vi "iPSread.vi"(8 "error in (no error)":errorcluster, 10 "iPSreadCtrl":T1=enum."Switch Heater Temp", 11 "VISA resource name":refnum<visa-resource-name>) -> (0 "error out":errorcluster, 1 "read buffer":string, 2 "number":dbl, 3 "VISA resource name out":refnum<visa-resource-name>)   [LabVIEW 2017]
uses:
  controls/iPSreadCtrl.ctl
  <vilib>/regexp/Match Regular Expression.xnode
panel:
  out "after match":string
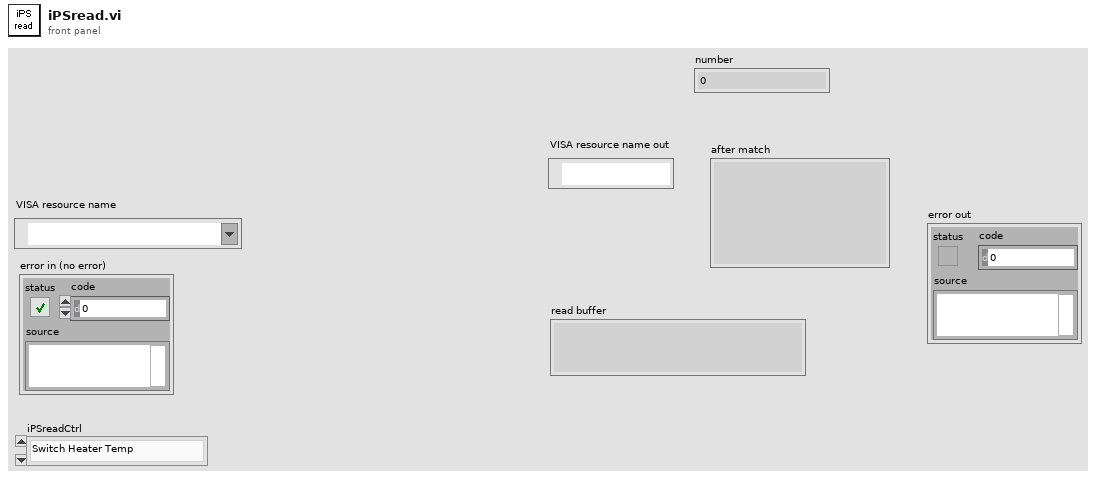
[diagram p1: front panel]
types:
  T1 = typedef "iPSreadCtrl.ctl" = enum16{"OutputField", "MagnetField", "Switch Heater Temp", "Field Rate", "Magnet Temp", "OutputVoltage"}
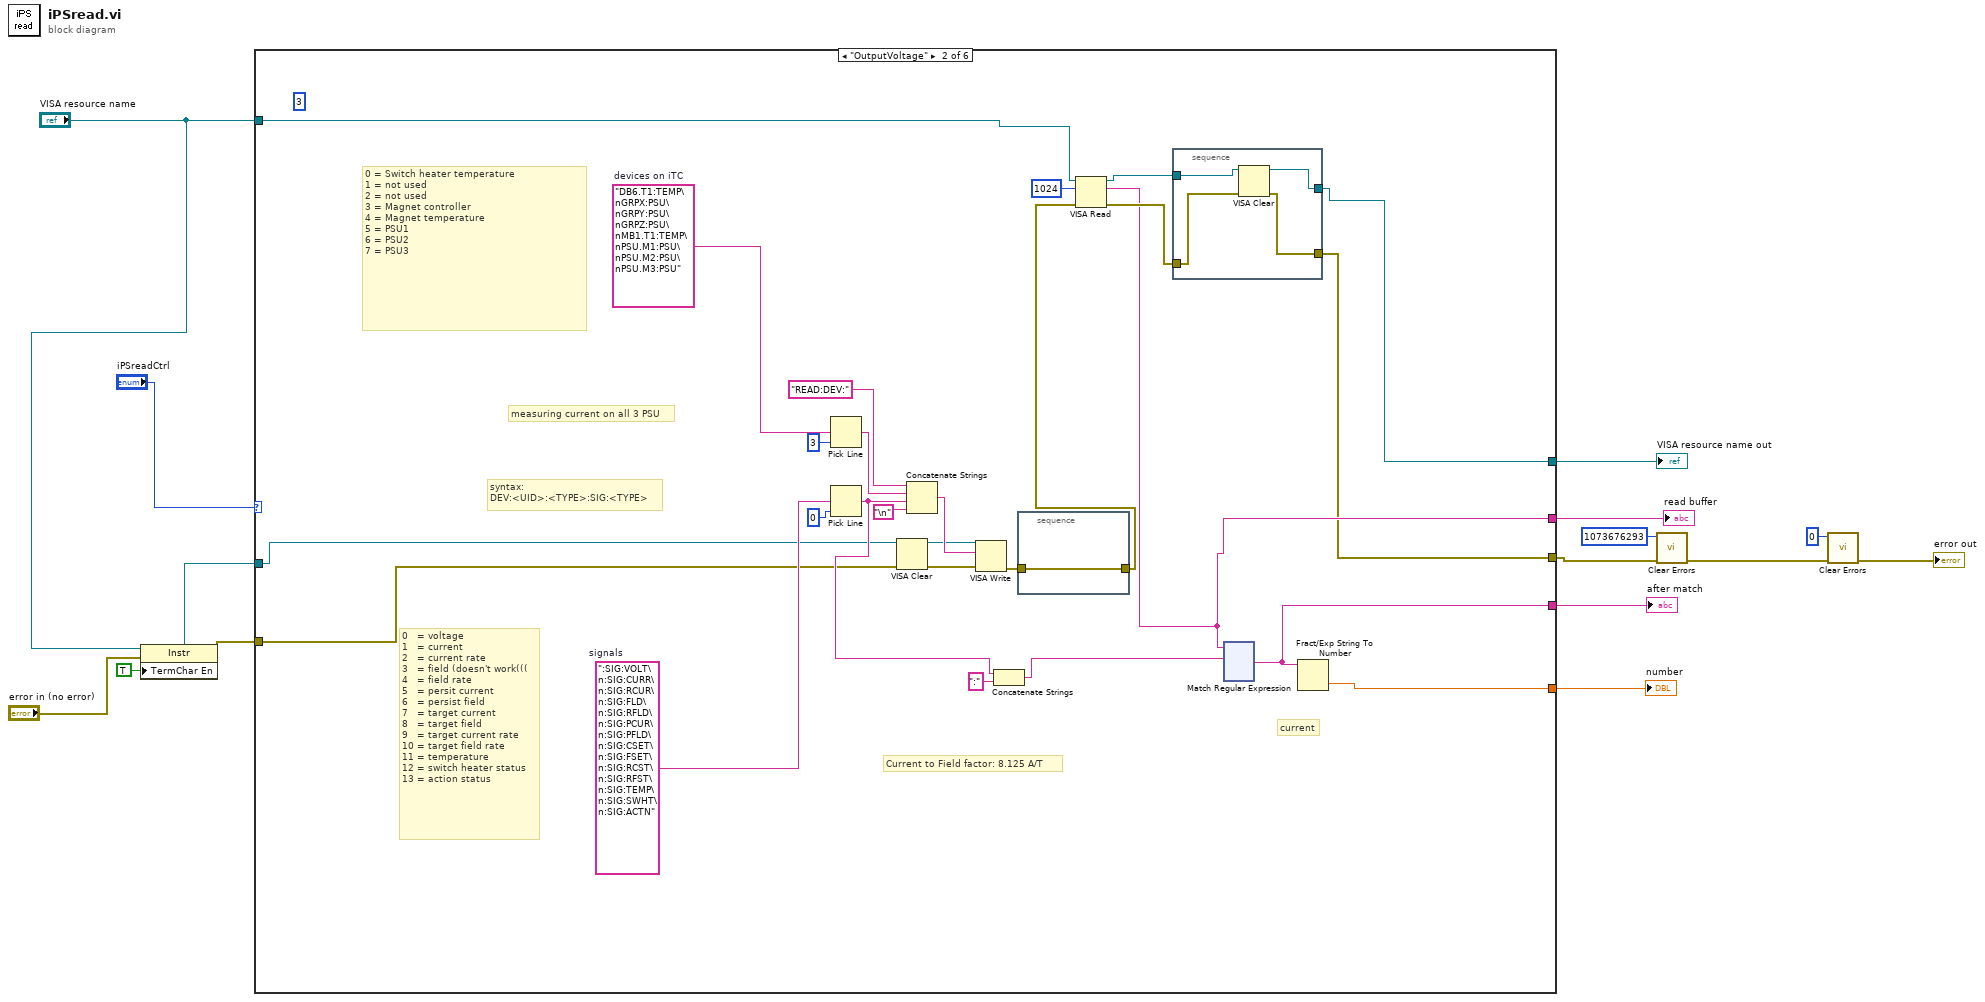
[diagram p0: block diagram]
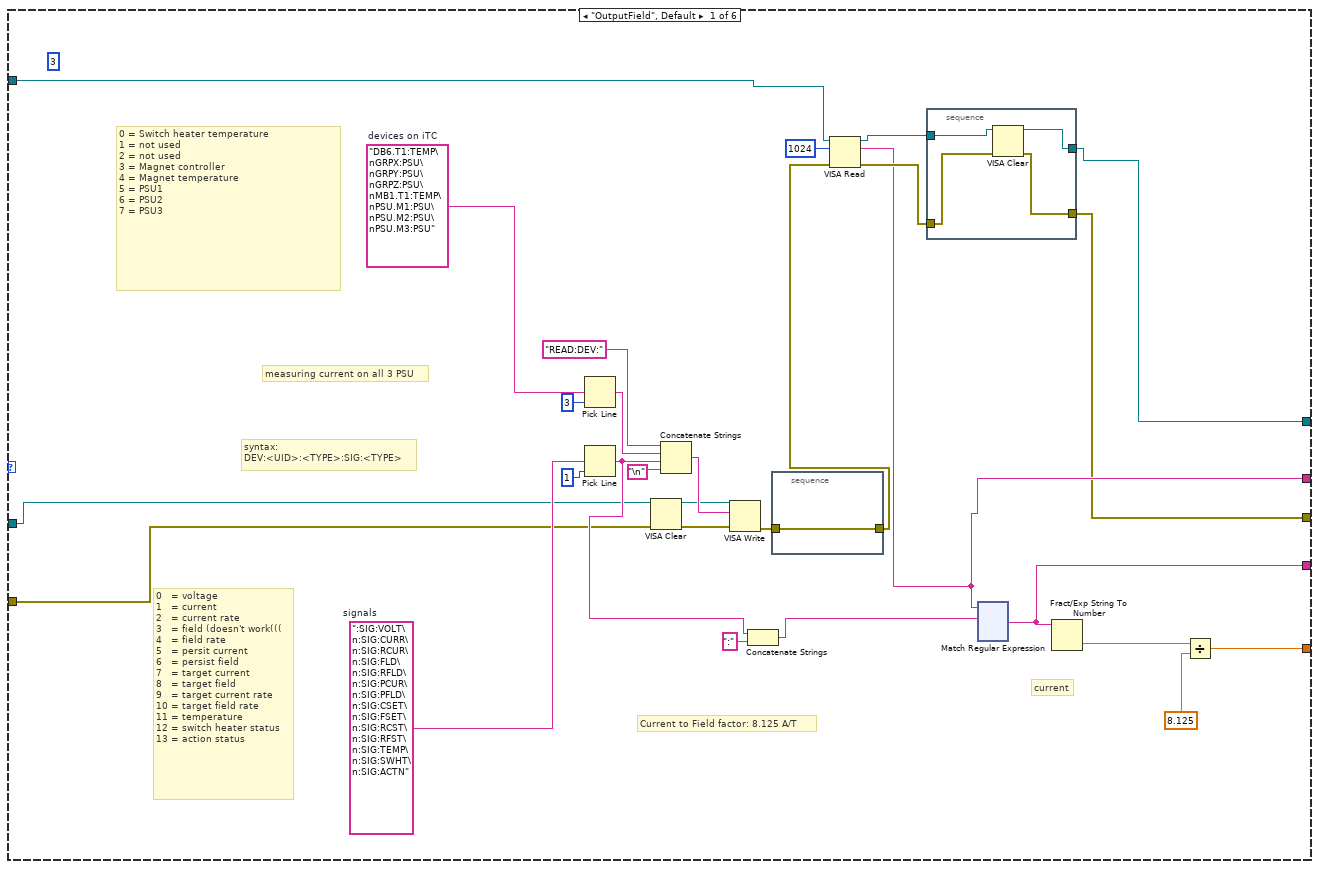
[diagram p2: hidden frame]
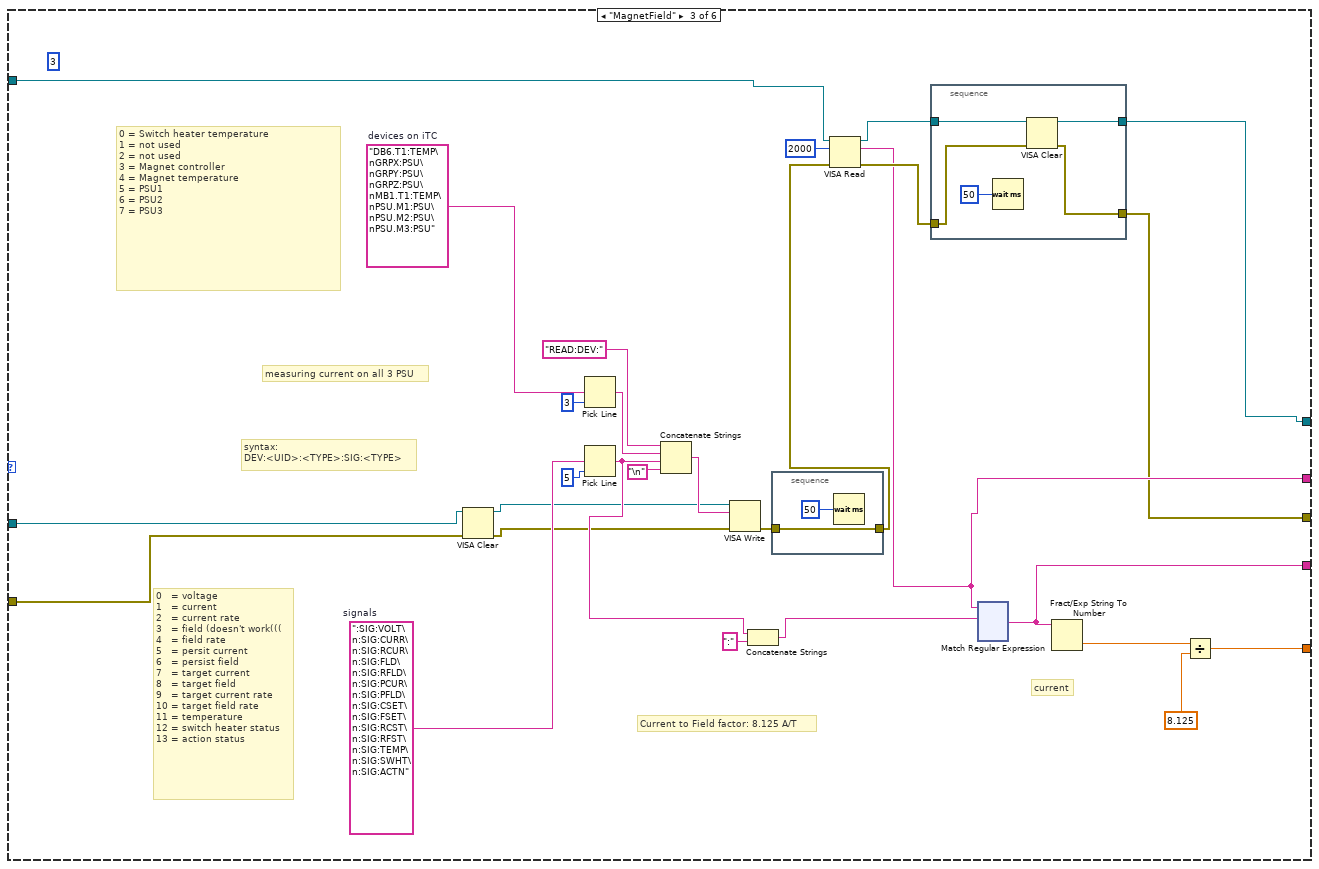
[diagram p3: hidden frame]
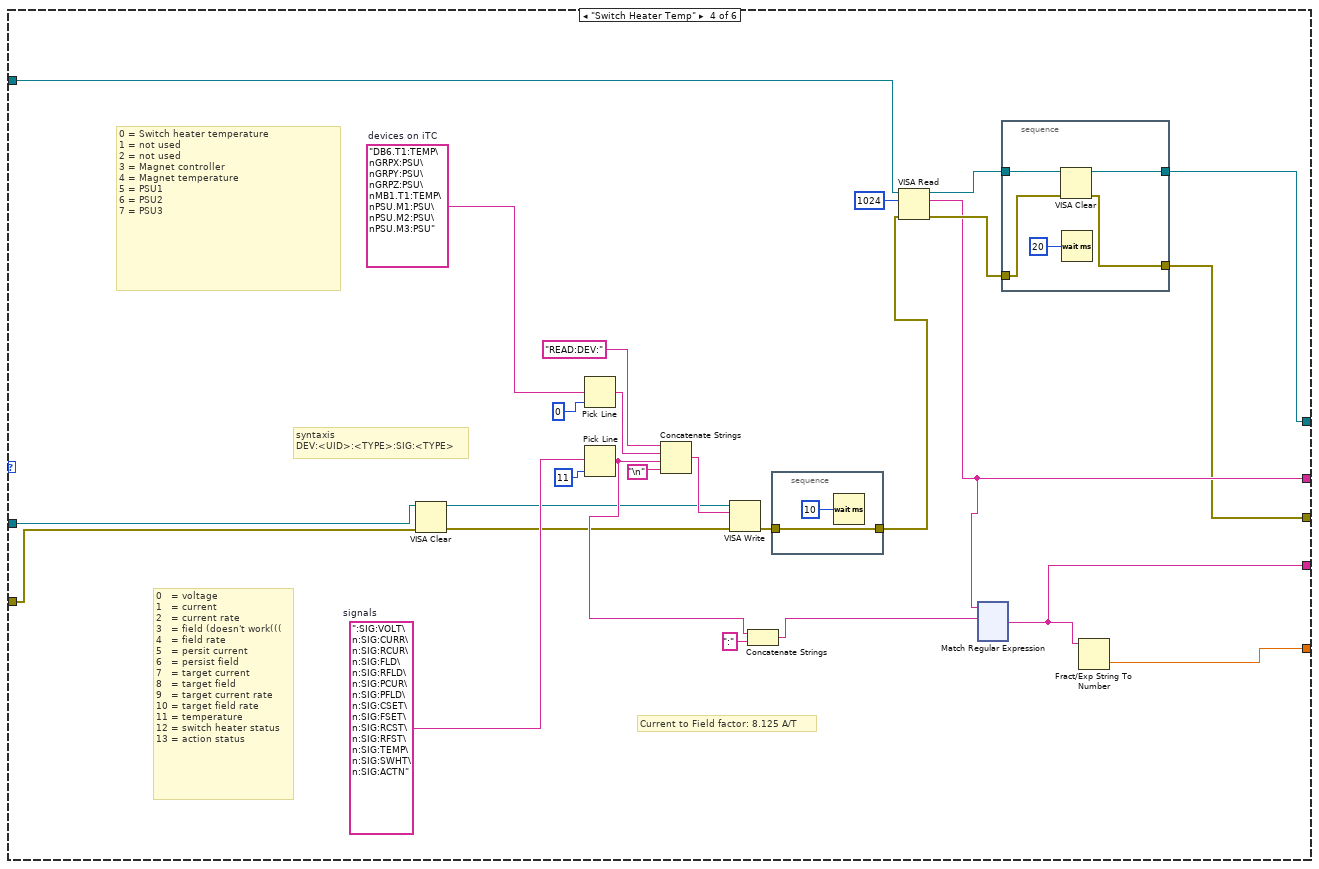
[diagram p4: hidden frame]
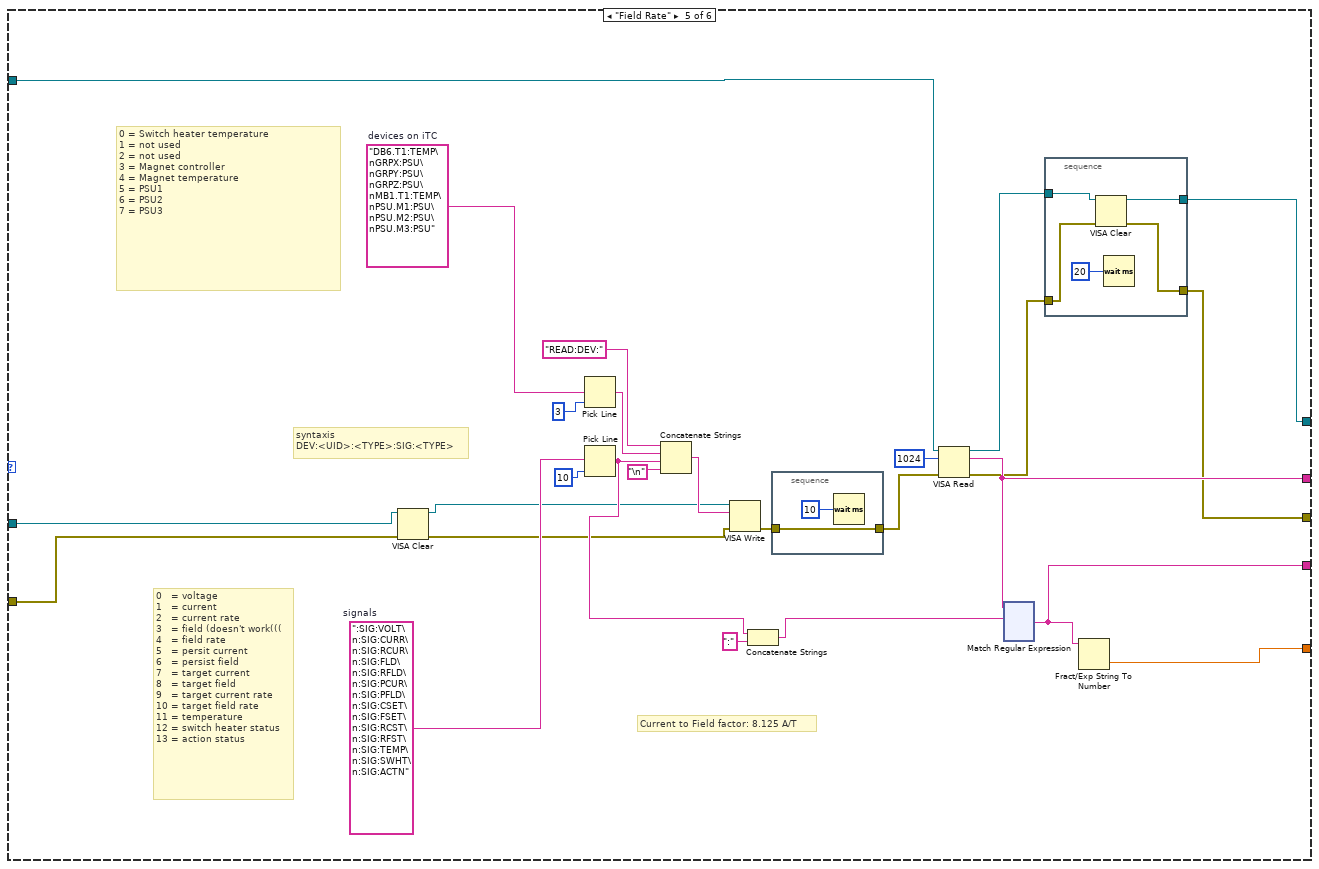
[diagram p5: hidden frame]
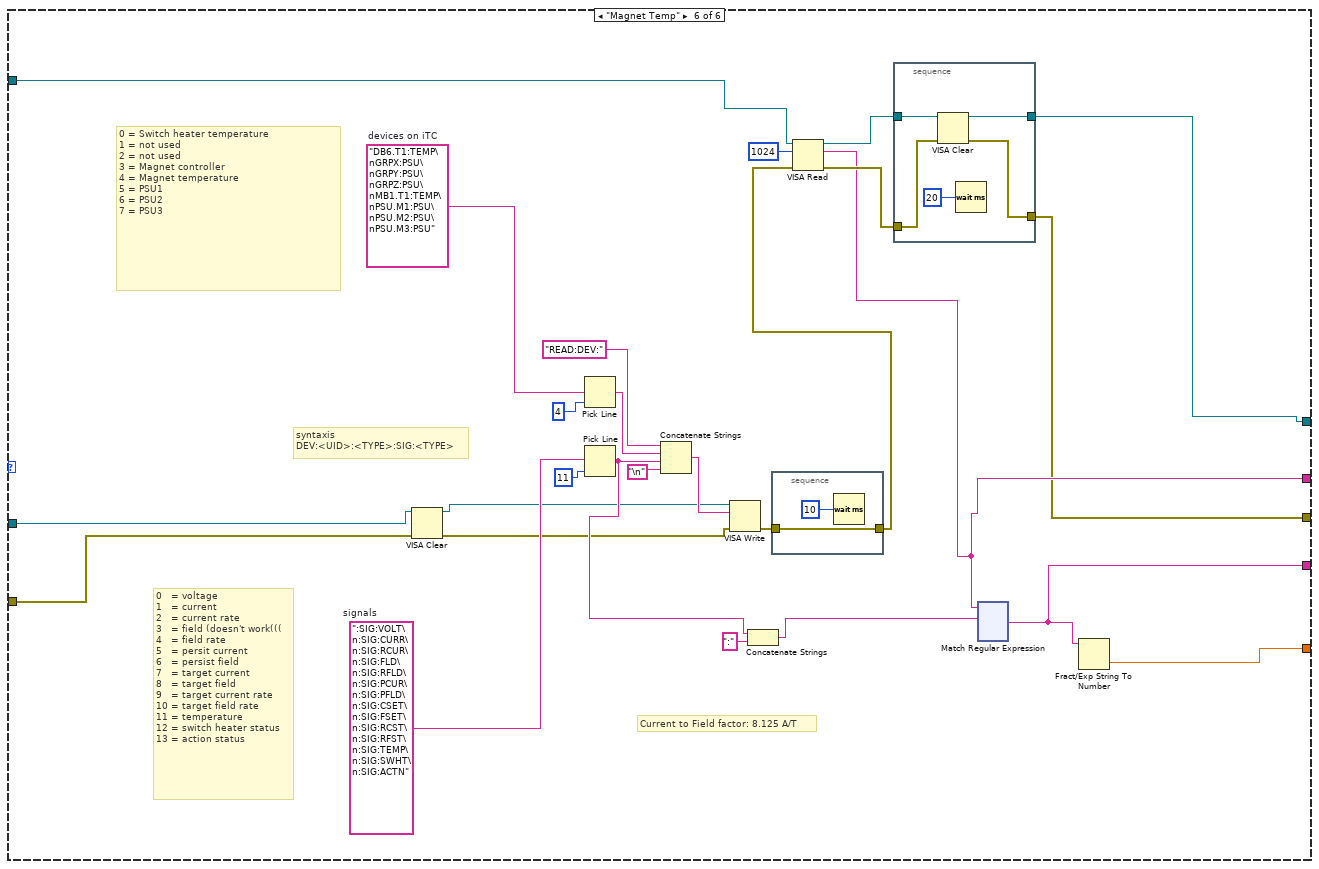
[diagram p6: hidden frame]
diagram:
  n1 = property class="Instr"(reference="VISA resource name", error in="error in (no error)", "TermChar En"=TRUE ("Message Based Settings:Termination Character Enable")) -> (reference out=w9:refnum<visa-resource-name>, error out=w7:errorcluster)
  n2 = case shown="\"OutputVoltage\"" "iPSreadCtrl" {
    tunnel: "VISA resource name" -> [w22 w167 w308 w454 w598 w745]
    tunnel: [w23 w168 w309 w455 w599 w742] -> w5
    tunnel: [w16 w161 w302 w449 w592 w737] -> w15
    tunnel: [w24 w169 w310 w457 w602 w743] -> w14
    tunnel: [w43 w185 w329 w463 w607 w751] -> w13
    tunnel: [w41 w160 w327 w462 w606 w750] -> w12
    tunnel: w7 -> [w20 w165 w304 w450 w596 w738]
    tunnel: w9 -> [w21 w166 w305 w451 w597 w739]
    frame "OutputField", Default {
      w35 = ":SIG:VOLT\n:SIG:CURR\n:SIG:RCUR\n:SIG:FLD\n:SIG:RFLD\n:SIG:PCUR\n:SIG:PFLD\n:SIG:CSET\n:SIG:FSET\n:SIG:RCST\n:SIG:RFST\n:SIG:TEMP\n:SIG:SWHT\n:SIG:ACTN"  # signals
      w40 = "DB6.T1:TEMP\nGRPX:PSU\nGRPY:PSU\nGRPZ:PSU\nMB1.T1:TEMP\nPSU.M1:PSU\nPSU.M2:PSU\nPSU.M3:PSU"  # devices on iTC
      (unwired) 3
      # "current"
      # "measuring current on all 3 PSU"
      # "Current to Field factor: 8.125 A/T"
      # "0 = Switch heater temperature\n1 = not used\n2 = not used\n3 = Magnet controller \n4 = Magnet temperature\n5 = PSU1 \n6 = PSU2\n7 = PSU3"
      # "0   = voltage\n1   = current\n2   = current rate\n3   = field (doesn't work(((\n4   = field rate\n5   = persit current\n6   = persist field\n7   = target current\n8   = target field\n9   = target current rate\n10 = target field rate \n11 = temperature\n12 = switch heater status\n13 = action status"
      # "syntax:\nDEV:<UID>:<TYPE>:SIG:<TYPE>"
      n3 = Pick Line(multi-line string=w40, line index=3) -> (output string=w37:string)  [unwired: 1 in]
      n4 = Pick Line(multi-line string=w35, line index=1) -> (output string=w33:string)  [unwired: 1 in]
      n5 = VISA Clear(VISA resource name=w21, error in (no error)=w20) -> (VISA resource name out=w19:refnum<visa-resource-name>, error out=w18:errorcluster)
      n6 = Concatenate Strings("READ:DEV:" ("write buffer"), w37, w33, "\n") -> (w31:string)
      n7 = VISA Write(VISA resource name=w19, write buffer=w31, error in (no error)=w18) -> (error out=w39:errorcluster)  [unwired: 2 out]
      n8 = Concatenate Strings(w33, ":" ("string")) -> (w32:string)
      n9 = stacked-sequence {
        tunnel: w39 -> [w159]
        tunnel: [w159] -> w25
        frame #0 {
        }
      }
      n10 = VISA Read(VISA resource name=w22, byte count=u32 1024, error in (no error)=w25) -> (VISA resource name out=w17:refnum<visa-resource-name>, read buffer=w24:string, error out=w26:errorcluster)  [unwired: 1 out]
      n11 = stacked-sequence {
        tunnel: [w46] -> w23
        tunnel: w26 -> [w45]
        tunnel: w17 -> [w44]
        tunnel: [w47] -> w16
        frame #0 {
          n12 = VISA Clear(VISA resource name=w44, error in (no error)=w45) -> (VISA resource name out=w47:refnum<visa-resource-name>, error out=w46:errorcluster)
        }
      }
      n13 = xnode "Match Regular Expression"("input string"=w24, "regular expression"=w32) -> ("after match"=w43:string)  [unwired: 4 in, 4 out]
      n14 = Fract/Exp String To Number(string=w43) -> (number=w28:dbl)  [unwired: 3 in, 1 out]
      n15 = Divide(x=w28, y=8.125) -> (x/y=w41:dbl)
    }
    frame "OutputVoltage" {
      w179 = ":SIG:VOLT\n:SIG:CURR\n:SIG:RCUR\n:SIG:FLD\n:SIG:RFLD\n:SIG:PCUR\n:SIG:PFLD\n:SIG:CSET\n:SIG:FSET\n:SIG:RCST\n:SIG:RFST\n:SIG:TEMP\n:SIG:SWHT\n:SIG:ACTN"  # signals
      w184 = "DB6.T1:TEMP\nGRPX:PSU\nGRPY:PSU\nGRPZ:PSU\nMB1.T1:TEMP\nPSU.M1:PSU\nPSU.M2:PSU\nPSU.M3:PSU"  # devices on iTC
      (unwired) 3
      # "current"
      # "measuring current on all 3 PSU"
      # "Current to Field factor: 8.125 A/T"
      # "0 = Switch heater temperature\n1 = not used\n2 = not used\n3 = Magnet controller \n4 = Magnet temperature\n5 = PSU1 \n6 = PSU2\n7 = PSU3"
      # "0   = voltage\n1   = current\n2   = current rate\n3   = field (doesn't work(((\n4   = field rate\n5   = persit current\n6   = persist field\n7   = target current\n8   = target field\n9   = target current rate\n10 = target field rate \n11 = temperature\n12 = switch heater status\n13 = action status"
      # "syntax:\nDEV:<UID>:<TYPE>:SIG:<TYPE>"
      n16 = Pick Line(multi-line string=w184, line index=3) -> (output string=w181:string)  [unwired: 1 in]
      n17 = Pick Line(multi-line string=w179, line index=0) -> (output string=w177:string)  [unwired: 1 in]
      n18 = VISA Clear(VISA resource name=w166, error in (no error)=w165) -> (VISA resource name out=w164:refnum<visa-resource-name>, error out=w163:errorcluster)
      n19 = Concatenate Strings("READ:DEV:" ("write buffer"), w181, w177, "\n") -> (w175:string)
      n20 = VISA Write(VISA resource name=w164, write buffer=w175, error in (no error)=w163) -> (error out=w183:errorcluster)  [unwired: 2 out]
      n21 = Concatenate Strings(w177, ":" ("string")) -> (w176:string)
      n22 = stacked-sequence {
        tunnel: w183 -> [w301]
        tunnel: [w301] -> w170
        frame #0 {
        }
      }
      n23 = VISA Read(VISA resource name=w167, byte count=u32 1024, error in (no error)=w170) -> (VISA resource name out=w162:refnum<visa-resource-name>, read buffer=w169:string, error out=w171:errorcluster)  [unwired: 1 out]
      n24 = stacked-sequence {
        tunnel: [w188] -> w168
        tunnel: w171 -> [w187]
        tunnel: w162 -> [w186]
        tunnel: [w189] -> w161
        frame #0 {
          n25 = VISA Clear(VISA resource name=w186, error in (no error)=w187) -> (VISA resource name out=w189:refnum<visa-resource-name>, error out=w188:errorcluster)
        }
      }
      n26 = xnode "Match Regular Expression"("input string"=w169, "regular expression"=w176) -> ("after match"=w185:string)  [unwired: 4 in, 4 out]
      n27 = Fract/Exp String To Number(string=w185) -> (number=w160:dbl)  [unwired: 3 in, 1 out]
    }
    frame "MagnetField" {
      w321 = ":SIG:VOLT\n:SIG:CURR\n:SIG:RCUR\n:SIG:FLD\n:SIG:RFLD\n:SIG:PCUR\n:SIG:PFLD\n:SIG:CSET\n:SIG:FSET\n:SIG:RCST\n:SIG:RFST\n:SIG:TEMP\n:SIG:SWHT\n:SIG:ACTN"  # signals
      w326 = "DB6.T1:TEMP\nGRPX:PSU\nGRPY:PSU\nGRPZ:PSU\nMB1.T1:TEMP\nPSU.M1:PSU\nPSU.M2:PSU\nPSU.M3:PSU"  # devices on iTC
      (unwired) 3
      # "current"
      # "measuring current on all 3 PSU"
      # "Current to Field factor: 8.125 A/T"
      # "0 = Switch heater temperature\n1 = not used\n2 = not used\n3 = Magnet controller \n4 = Magnet temperature\n5 = PSU1 \n6 = PSU2\n7 = PSU3"
      # "0   = voltage\n1   = current\n2   = current rate\n3   = field (doesn't work(((\n4   = field rate\n5   = persit current\n6   = persist field\n7   = target current\n8   = target field\n9   = target current rate\n10 = target field rate \n11 = temperature\n12 = switch heater status\n13 = action status"
      # "syntax:\nDEV:<UID>:<TYPE>:SIG:<TYPE>"
      n28 = VISA Clear(VISA resource name=w305, error in (no error)=w304) -> (VISA resource name out=w307:refnum<visa-resource-name>, error out=w306:errorcluster)
      n29 = Pick Line(multi-line string=w326, line index=3) -> (output string=w323:string)  [unwired: 1 in]
      n30 = Pick Line(multi-line string=w321, line index=5) -> (output string=w319:string)  [unwired: 1 in]
      n31 = Concatenate Strings("READ:DEV:" ("write buffer"), w323, w319, "\n") -> (w317:string)
      n32 = VISA Write(VISA resource name=w307, write buffer=w317, error in (no error)=w306) -> (error out=w325:errorcluster)  [unwired: 2 out]
      n33 = Concatenate Strings(w319, ":" ("string")) -> (w318:string)
      n34 = stacked-sequence {
        tunnel: w325 -> [w447]
        tunnel: [w447] -> w311
        frame #0 {
          n35 = Wait (ms)(milliseconds to wait=u32 50) -> ()  [unwired: 1 out]
        }
      }
      n36 = VISA Read(VISA resource name=w308, byte count=u32 2000, error in (no error)=w311) -> (VISA resource name out=w303:refnum<visa-resource-name>, read buffer=w310:string, error out=w312:errorcluster)  [unwired: 1 out]
      n37 = stacked-sequence {
        tunnel: [w331] -> w309
        tunnel: w312 -> [w330]
        tunnel: w303 -> [w333]
        tunnel: [w332] -> w302
        frame #0 {
          n38 = Wait (ms)(milliseconds to wait=u32 50) -> ()  [unwired: 1 out]
          n39 = VISA Clear(VISA resource name=w333, error in (no error)=w330) -> (VISA resource name out=w332:refnum<visa-resource-name>, error out=w331:errorcluster)
        }
      }
      n40 = xnode "Match Regular Expression"("input string"=w310, "regular expression"=w318) -> ("after match"=w329:string)  [unwired: 4 in, 4 out]
      n41 = Fract/Exp String To Number(string=w329) -> (number=w314:dbl)  [unwired: 3 in, 1 out]
      n42 = Divide(x=w314, y=8.125) -> (x/y=w327:dbl)
    }
    frame "Switch Heater Temp" {
      w468 = ":SIG:VOLT\n:SIG:CURR\n:SIG:RCUR\n:SIG:FLD\n:SIG:RFLD\n:SIG:PCUR\n:SIG:PFLD\n:SIG:CSET\n:SIG:FSET\n:SIG:RCST\n:SIG:RFST\n:SIG:TEMP\n:SIG:SWHT\n:SIG:ACTN"  # signals
      w473 = "DB6.T1:TEMP\nGRPX:PSU\nGRPY:PSU\nGRPZ:PSU\nMB1.T1:TEMP\nPSU.M1:PSU\nPSU.M2:PSU\nPSU.M3:PSU"  # devices on iTC
      # "Current to Field factor: 8.125 A/T"
      # "0 = Switch heater temperature\n1 = not used\n2 = not used\n3 = Magnet controller \n4 = Magnet temperature\n5 = PSU1 \n6 = PSU2\n7 = PSU3"
      # "0   = voltage\n1   = current\n2   = current rate\n3   = field (doesn't work(((\n4   = field rate\n5   = persit current\n6   = persist field\n7   = target current\n8   = target field\n9   = target current rate\n10 = target field rate \n11 = temperature\n12 = switch heater status\n13 = action status"
      # "syntaxis\nDEV:<UID>:<TYPE>:SIG:<TYPE>"
      n43 = VISA Clear(VISA resource name=w451, error in (no error)=w450) -> (VISA resource name out=w453:refnum<visa-resource-name>, error out=w452:errorcluster)
      n44 = Pick Line(multi-line string=w473, line index=0) -> (output string=w470:string)  [unwired: 1 in]
      n45 = Pick Line(multi-line string=w468, line index=11) -> (output string=w466:string)  [unwired: 1 in]
      n46 = Concatenate Strings("READ:DEV:" ("write buffer"), w470, w466, "\n") -> (w464:string)
      n47 = VISA Write(VISA resource name=w453, write buffer=w464, error in (no error)=w452) -> (error out=w472:errorcluster)  [unwired: 2 out]
      n48 = Concatenate Strings(w466, ":" ("string")) -> (w465:string)
      n49 = stacked-sequence {
        tunnel: w472 -> [w591]
        tunnel: [w591] -> w456
        frame #0 {
          n50 = Wait (ms)(milliseconds to wait=u32 10) -> ()  [unwired: 1 out]
        }
      }
      n51 = VISA Read(VISA resource name=w454, byte count=u32 1024, error in (no error)=w456) -> (VISA resource name out=w448:refnum<visa-resource-name>, read buffer=w457:string, error out=w458:errorcluster)  [unwired: 1 out]
      n52 = xnode "Match Regular Expression"("input string"=w457, "regular expression"=w465) -> ("after match"=w463:string)  [unwired: 4 in, 4 out]
      n53 = stacked-sequence {
        tunnel: [w477] -> w455
        tunnel: w458 -> [w476]
        tunnel: [w475] -> w449
        tunnel: w448 -> [w474]
        frame #0 {
          n54 = VISA Clear(VISA resource name=w474, error in (no error)=w476) -> (VISA resource name out=w475:refnum<visa-resource-name>, error out=w477:errorcluster)
          n55 = Wait (ms)(milliseconds to wait=u32 20) -> ()  [unwired: 1 out]
        }
      }
      n56 = Fract/Exp String To Number(string=w463) -> (number=w462:dbl)  [unwired: 3 in, 1 out]
    }
    frame "Field Rate" {
      w612 = ":SIG:VOLT\n:SIG:CURR\n:SIG:RCUR\n:SIG:FLD\n:SIG:RFLD\n:SIG:PCUR\n:SIG:PFLD\n:SIG:CSET\n:SIG:FSET\n:SIG:RCST\n:SIG:RFST\n:SIG:TEMP\n:SIG:SWHT\n:SIG:ACTN"  # signals
      w617 = "DB6.T1:TEMP\nGRPX:PSU\nGRPY:PSU\nGRPZ:PSU\nMB1.T1:TEMP\nPSU.M1:PSU\nPSU.M2:PSU\nPSU.M3:PSU"  # devices on iTC
      # "Current to Field factor: 8.125 A/T"
      # "0 = Switch heater temperature\n1 = not used\n2 = not used\n3 = Magnet controller \n4 = Magnet temperature\n5 = PSU1 \n6 = PSU2\n7 = PSU3"
      # "0   = voltage\n1   = current\n2   = current rate\n3   = field (doesn't work(((\n4   = field rate\n5   = persit current\n6   = persist field\n7   = target current\n8   = target field\n9   = target current rate\n10 = target field rate \n11 = temperature\n12 = switch heater status\n13 = action status"
      # "syntaxis\nDEV:<UID>:<TYPE>:SIG:<TYPE>"
      n57 = VISA Clear(VISA resource name=w597, error in (no error)=w596) -> (VISA resource name out=w595:refnum<visa-resource-name>, error out=w594:errorcluster)
      n58 = Pick Line(multi-line string=w617, line index=3) -> (output string=w614:string)  [unwired: 1 in]
      n59 = Pick Line(multi-line string=w612, line index=10) -> (output string=w610:string)  [unwired: 1 in]
      n60 = Concatenate Strings("READ:DEV:" ("write buffer"), w614, w610, "\n") -> (w608:string)
      n61 = VISA Write(VISA resource name=w595, write buffer=w608, error in (no error)=w594) -> (error out=w616:errorcluster)  [unwired: 2 out]
      n62 = Concatenate Strings(w610, ":" ("string")) -> (w609:string)
      n63 = stacked-sequence {
        tunnel: w616 -> [w735]
        tunnel: [w735] -> w601
        frame #0 {
          n64 = Wait (ms)(milliseconds to wait=u32 10) -> ()  [unwired: 1 out]
        }
      }
      n65 = VISA Read(VISA resource name=w598, byte count=u32 1024, error in (no error)=w601) -> (VISA resource name out=w593:refnum<visa-resource-name>, read buffer=w602:string, error out=w600:errorcluster)  [unwired: 1 out]
      n66 = xnode "Match Regular Expression"("input string"=w602, "regular expression"=w609) -> ("after match"=w607:string)  [unwired: 4 in, 4 out]
      n67 = stacked-sequence {
        tunnel: [w621] -> w599
        tunnel: w600 -> [w620]
        tunnel: w593 -> [w619]
        tunnel: [w618] -> w592
        frame #0 {
          n68 = VISA Clear(VISA resource name=w619, error in (no error)=w620) -> (VISA resource name out=w618:refnum<visa-resource-name>, error out=w621:errorcluster)
          n69 = Wait (ms)(milliseconds to wait=u32 20) -> ()  [unwired: 1 out]
        }
      }
      n70 = Fract/Exp String To Number(string=w607) -> (number=w606:dbl)  [unwired: 3 in, 1 out]
    }
    frame "Magnet Temp" {
      w756 = ":SIG:VOLT\n:SIG:CURR\n:SIG:RCUR\n:SIG:FLD\n:SIG:RFLD\n:SIG:PCUR\n:SIG:PFLD\n:SIG:CSET\n:SIG:FSET\n:SIG:RCST\n:SIG:RFST\n:SIG:TEMP\n:SIG:SWHT\n:SIG:ACTN"  # signals
      w761 = "DB6.T1:TEMP\nGRPX:PSU\nGRPY:PSU\nGRPZ:PSU\nMB1.T1:TEMP\nPSU.M1:PSU\nPSU.M2:PSU\nPSU.M3:PSU"  # devices on iTC
      # "Current to Field factor: 8.125 A/T"
      # "0 = Switch heater temperature\n1 = not used\n2 = not used\n3 = Magnet controller \n4 = Magnet temperature\n5 = PSU1 \n6 = PSU2\n7 = PSU3"
      # "0   = voltage\n1   = current\n2   = current rate\n3   = field (doesn't work(((\n4   = field rate\n5   = persit current\n6   = persist field\n7   = target current\n8   = target field\n9   = target current rate\n10 = target field rate \n11 = temperature\n12 = switch heater status\n13 = action status"
      # "syntaxis\nDEV:<UID>:<TYPE>:SIG:<TYPE>"
      n71 = VISA Clear(VISA resource name=w739, error in (no error)=w738) -> (VISA resource name out=w741:refnum<visa-resource-name>, error out=w740:errorcluster)
      n72 = Pick Line(multi-line string=w761, line index=4) -> (output string=w758:string)  [unwired: 1 in]
      n73 = Pick Line(multi-line string=w756, line index=11) -> (output string=w754:string)  [unwired: 1 in]
      n74 = Concatenate Strings("READ:DEV:" ("write buffer"), w758, w754, "\n") -> (w752:string)
      n75 = VISA Write(VISA resource name=w741, write buffer=w752, error in (no error)=w740) -> (error out=w760:errorcluster)  [unwired: 2 out]
      n76 = Concatenate Strings(w754, ":" ("string")) -> (w753:string)
      n77 = stacked-sequence {
        tunnel: w760 -> [w879]
        tunnel: [w879] -> w744
        frame #0 {
          n78 = Wait (ms)(milliseconds to wait=u32 10) -> ()  [unwired: 1 out]
        }
      }
      n79 = VISA Read(VISA resource name=w745, byte count=u32 1024, error in (no error)=w744) -> (VISA resource name out=w736:refnum<visa-resource-name>, read buffer=w743:string, error out=w746:errorcluster)  [unwired: 1 out]
      n80 = stacked-sequence {
        tunnel: [w765] -> w742
        tunnel: w746 -> [w764]
        tunnel: [w763] -> w737
        tunnel: w736 -> [w762]
        frame #0 {
          n81 = VISA Clear(VISA resource name=w762, error in (no error)=w764) -> (VISA resource name out=w763:refnum<visa-resource-name>, error out=w765:errorcluster)
          n82 = Wait (ms)(milliseconds to wait=u32 20) -> ()  [unwired: 1 out]
        }
      }
      n83 = xnode "Match Regular Expression"("input string"=w743, "regular expression"=w753) -> ("after match"=w751:string)  [unwired: 4 in, 4 out]
      n84 = Fract/Exp String To Number(string=w751) -> (number=w750:dbl)  [unwired: 3 in, 1 out]
    }
  }
  "read buffer" <- w14
  "VISA resource name out" <- w15
  "after match" <- w13
  "number" <- w12
  n85 = call <vilib>:"Clear Errors.vi"("error in (no error)"=w5, "specific error code to clear (0: all)"=1073676293) -> ("error out"=w3:errorcluster)  [unwired: 4 in, 1 out]
  n86 = call <vilib>:"Clear Errors.vi"("error in (no error)"=w3, "specific error code to clear (0: all)"=0) -> ("error out"=→"error out":errorcluster)  [unwired: 4 in, 1 out]
